vi "Test Flip ARGB.vi"(8 "error in (no error)":errorcluster, 11 "Test Case In":refnum<class "Image.lvclass">) -> (0 "error out":errorcluster, 3 "Test Case Out":refnum<class "Image.lvclass">)   [LabVIEW 2020, in "g_ar_toolkit.test.lvlib" / "Image.lvclass"]
uses:
  Image.lvclass
  C:/Program Files (x86)/National Instruments/LabVIEW 2020/vi.lib/Astemes/LUnit/Test Case.lvclass
  g_ar_toolkit.image/Flip Mode.ctl
  g_ar_toolkit.common/Image Size (Integer).ctl
  <vilib>/Astemes/LUnit/Test Case.lvclass/Test Case.ctl
  g_ar_toolkit.image/CreateEmptyImageARGB.vi
  g_ar_toolkit.image/FlipARGB.vi
  4993e8ee-a06a-463a-9684-69129f64d5ce.vi
  g_ar_toolkit.image/Copy Array to Image.vi
  g_ar_toolkit.image/CopyArrayToImageARGB.vi
  g_ar_toolkit.image/CreateEmptyImageARGB.vi/3321fa97-f432-4e1e-8db9-a0df79aed21b.vi
  g_ar_toolkit.image/FlipARGB.vi/348de330-10c9-445f-8d54-7780e9118077.vi
  <vilib>/Astemes/LUnit/Append Pass Result.vi
  <vilib>/Astemes/LUnit/Append Fail Result.vi
  <vilib>/Astemes/LUnit/Describe Comparison.vi
  <vilib>/Astemes/LUnit/Compare Variants.vi
  g_ar_toolkit.image/CopyArrayToImageARGB.vi/26c70cee-9332-41f4-9755-08948a885cbe.vi
  <vilib>/Astemes/LUnit/Run In UI.vi
  <vilib>/Utility/error.llb/Clear Errors.vi
  g_ar_toolkit.image/ARGBColourToU32.vi
  g_ar_toolkit.common/Module Path.vi
  <vilib>/Utility/error.llb/Error Cluster From Error Code.vi
  <vilib>/picture/pixmap.llb/Flatten Pixmap.vi
  <vilib>/Astemes/LUnit/Describe Variant.vi
  Image.lvclass/Image.ctl
  g_ar_toolkit.image/g_ar_toolkit.image.lvlib
  g_ar_toolkit.common/g_ar_toolkit.common.lvlib
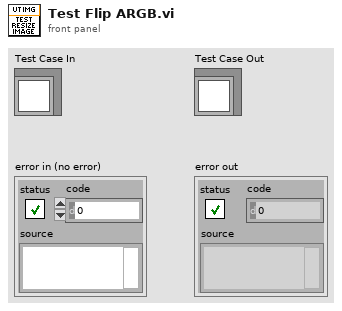
[diagram p1: front panel]
types:
  T1 = typedef "g_ar_toolkit.common.lvlib/Image Size (Integer).ctl" = cluster{"Width":u16, "Height":u16}
  T2 = typedef "g_ar_toolkit.image.lvlib/Flip Mode.ctl" = enum8{"X-Axis", "Y-Axis", "X and Y Axes"}
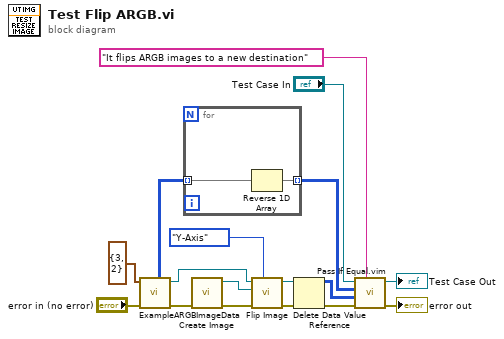
[diagram p0: block diagram]
diagram:
  n1 = call "ExampleARGBImageData.vi"("error in (no error)"="error in (no error)", "Image Size"=T1 {"Width"=3, "Height"=2}) -> ("error out"=w5:errorcluster, "Data Value Reference out"=w3:refnum<data-value>, "ARGB Array Data"=w1:u32[][])  [unwired: 6 in, 1 out]
  n2 = for {
    tunnel: [w19] -> w7 mode=indexing
    tunnel: w1 -> [w18] mode=indexing
    n3 = Reverse 1D Array(array=w18) -> (reversed array=w19:u32[])
  }
  n4 = call-poly "Create Image.vi"("error in (no error)"=w5) -> ("error out"=w10:errorcluster, "New ARGB Image"=w8:refnum<data-value>)  [unwired: 9 in]
  n5 = call-poly "Flip Image.vi"("Flip Mode (Default: Y-Axis)"=Flip_Mode."Y-Axis" ("Flip Mode (Default: X-Axis)"), "error in (no error)"=w10, "ARGB Destination Image"=w8, "ARGB Source Image"=w3) -> ("error out"=w11:errorcluster, "ARGB  Destination Image (duplicate)"=w12:refnum<data-value>)  [unwired: 6 in]
  n6 = Delete Data Value Reference(data value reference=w12, error in=w11) -> (data value=w9:u32[][], error out=w14:errorcluster)
  n7 = call "Pass If Equal.vim"("Description"="It flips ARGB images to a new destination", "error in (no error)"=w14, "Actual"=w9, "Expected"=w7, "LUnit Test Case In"="Test Case In") -> ("error out"=→"error out":errorcluster, "LUnit Test Case Out"=→"Test Case Out":refnum<class "Image.lvclass">)  [unwired: 5 in]
